vi "Before Hook.vi"(7 "Hooks Search Path":T1, 8 "Error In":errorcluster, 11 "Hook VI":refnum<vi>) -> (0 "Error Out":errorcluster, 3 "Hook VI":path)   [LabVIEW 2018, in "Tests.lvlib" / "Toolkit.lvlib" / "Integration.lvlib"]
uses:
  Integration.lvlib
  Hook Search Paths.ctl
  src/Toolkit/Toolkit.lvlib
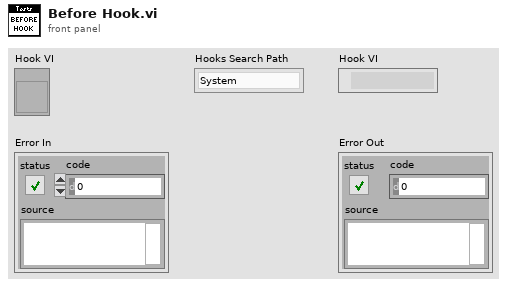
[diagram p1: front panel]
types:
  T1 = typedef "Tests.lvlib/Toolkit.lvlib/Integration.lvlib/Hook Search Paths.ctl" = enum32{"System", "User", "Project (Hidden)", "Project (Visible)"}
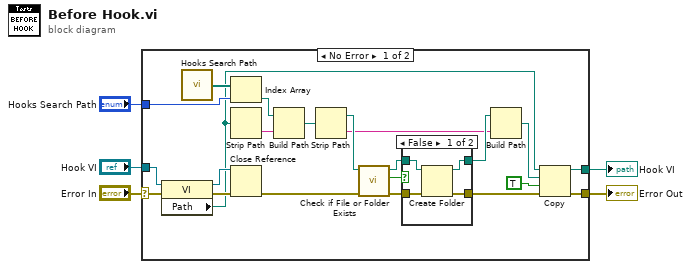
[diagram p0: block diagram]
diagram:
  n1 = case shown="No Error" "Error In" {
    selector: "Error In" -> [w20 w34]
    tunnel: [w27 _] -> w5
    tunnel: [w26 w34] -> w4
    tunnel: "Hooks Search Path" -> [w25 _]
    tunnel: "Hook VI" -> [w21 _]
    frame No Error {
      n2 = property class="VI"(reference=w21, error in=w20) -> (reference out=w23:refnum<vi>, error out=w22:errorcluster, "Path"=w6:path)
      n3 = call "Hooks Search Path.vi"() -> ("Hooks Search Path"=w24:path[])  [unwired: 1 in]
      n4 = Index Array(array=w24, index=w25) -> (element=w13:path)
      n5 = Strip Path(path=w6) -> (name=w8:string)  [unwired: 1 out]
      n6 = Close Reference(reference=w23, error in (no error)=w22) -> (error out=w7:errorcluster)
      n7 = Build Path(base path=w13, name or relative path=w8) -> (appended path=w15:path)
      n8 = Strip Path(path=w15) -> (stripped path=w14:path, name=w11:string)
      n9 = call <vilib>:"Check if File or Folder Exists.vi"("error in (no error)"=w7, "path"=w14) -> ("error out"=w17:errorcluster, "file or folder exists?"=w19:bool, "dup path"=w18:path)  [unwired: 7 in]
      n10 = case shown="False" w19 {
        tunnel: w18 -> [w31 w33]
        tunnel: w17 -> [w30 w32]
        tunnel: [w29 w33] -> w12
        tunnel: [w28 w32] -> w10
        frame False {
          n11 = Create Folder(path (use dialog)=w31, error in=w30) -> (created path=w29:path, error out=w28:errorcluster)  [unwired: 1 in, 1 out]
        }
        frame True {
        }
      }
      n12 = Build Path(base path=w12, name or relative path=w11) -> (appended path=w9:path)
      n13 = Copy(8:w10, 9:TRUE ("overwrite (F)"), 10:w9, 11:w6) -> (0:w26:errorcluster, 3:w27:path)  [unwired: 1 in, 1 out]
    }
    frame Error {
    }
  }
  "Hook VI" <- w5
  "Error Out" <- w4
